vi "Inst_CNT90.vi"(8 "error in":errorcluster, 10 "All Message Queues in":T2, 11 "Prueba031 in":refnum<class "Prueba031.lvclass">) -> (0 "error out":errorcluster)   [LabVIEW 2019, in "Prueba031.lvclass"]
uses:
  Prueba031.lvclass
  QMH/Message Queue/All Message Queues.ctl
  QMH/Message Queue/Message Cluster.ctl
  Prueba031.lvclass/Prueba031.ctl
  <vilib>/Utility/error.llb/Error Cluster From Error Code.vi
  QMH/Message Queue/Enqueue Message (Single).vi
  <vilib>/ErrorRing/Error Ring.xnode
  QMH/Message Queue/Message Queue.lvlib
  Instrumento/CNT90/CNT90.lvclass
panel:
  out "elements":T1[](array[typedef])
  out "# elements in queue":i32
  out "K_iter":i32
  out "All States":string[](array[string])
  out "Actual State":string
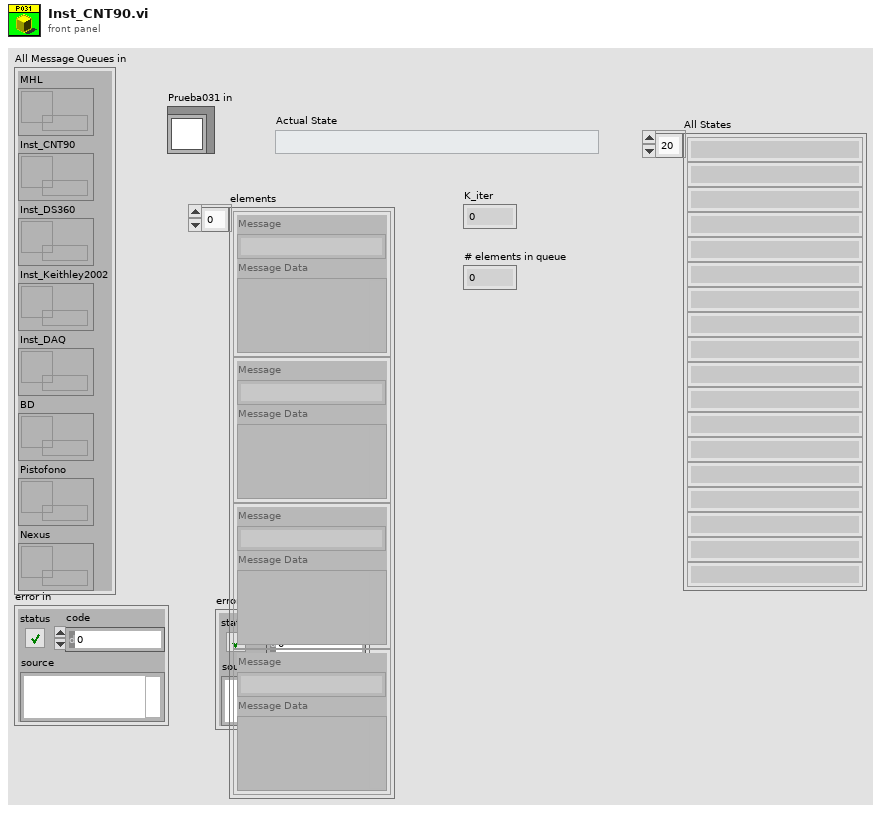
[diagram p1: front panel]
types:
  T1 = typedef "Message Queue.lvlib/Message Cluster.ctl" = cluster{"Message":string, "Message Data":variant}
  T2 = typedef "Message Queue.lvlib/All Message Queues.ctl" = cluster{"MHL":refnum<queue>, "Inst_CNT90":refnum<queue>, "Inst_DS360":refnum<queue>, "Inst_Keithley2002":refnum<queue>, "Inst_DAQ":refnum<queue>, "BD":refnum<queue>, "Pistofono":refnum<queue>, "Nexus":refnum<queue>}
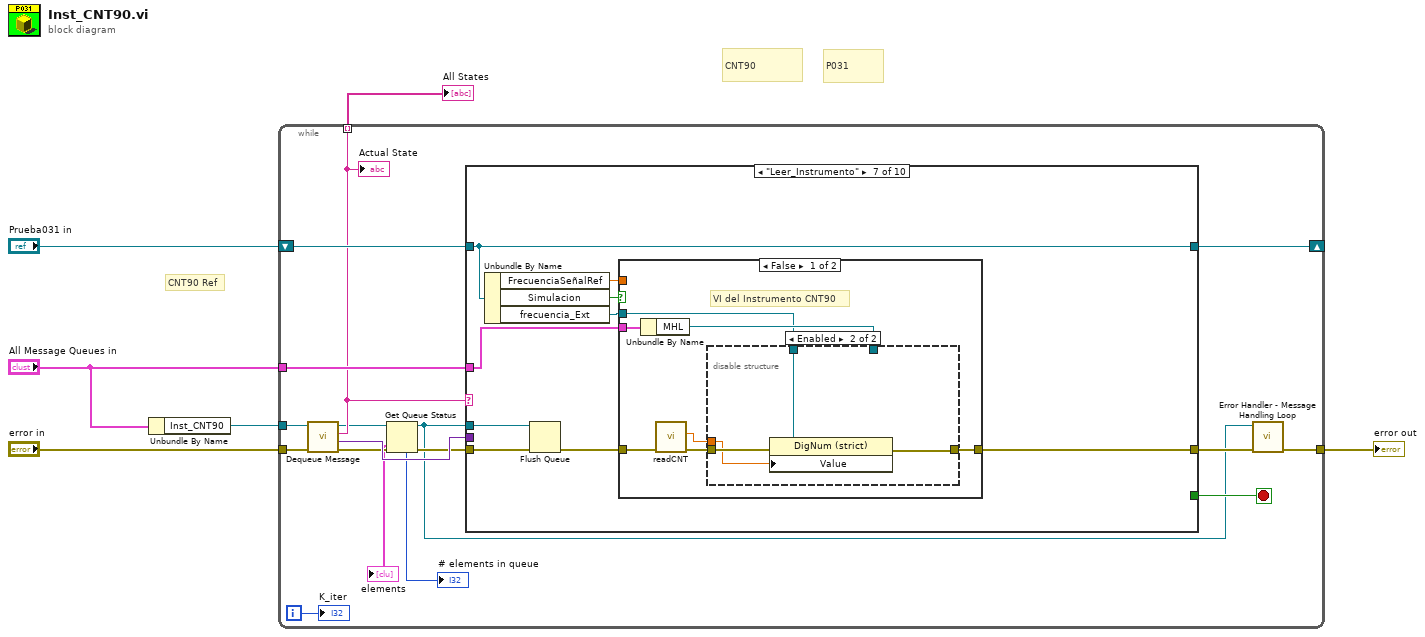
[diagram p0: block diagram]
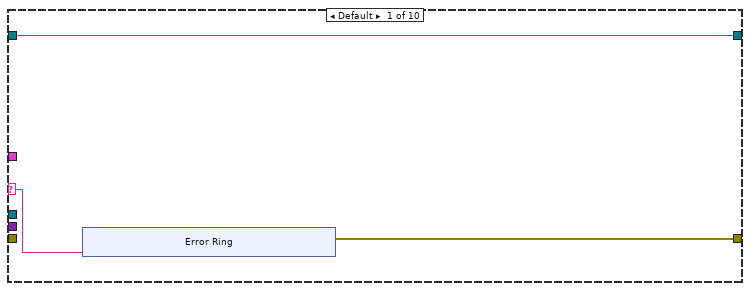
[diagram p2: hidden frame]
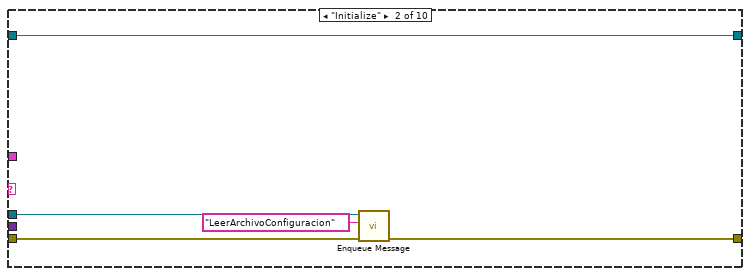
[diagram p3: hidden frame]
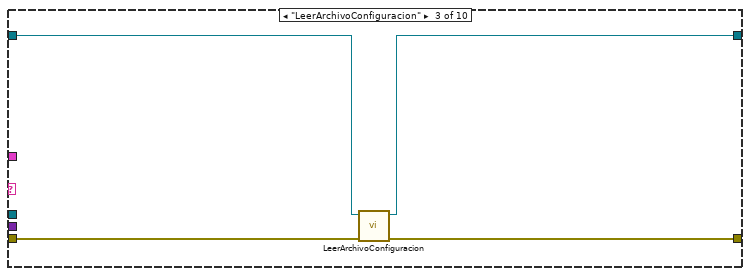
[diagram p4: hidden frame]
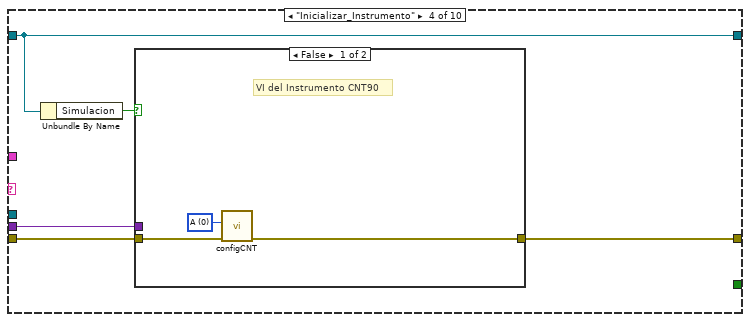
[diagram p5: hidden frame]
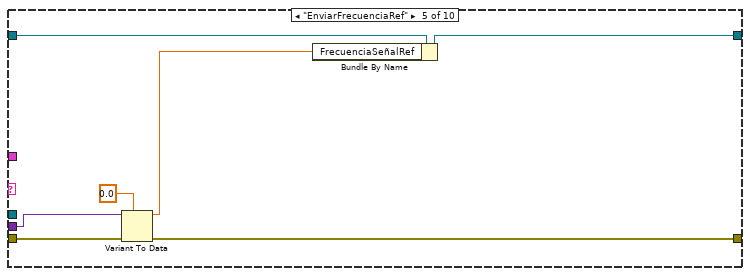
[diagram p7: hidden frame]
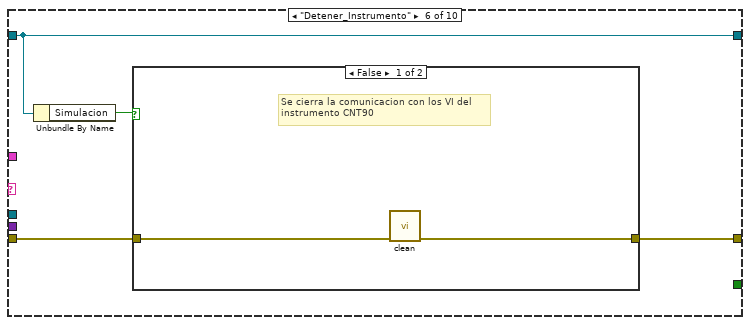
[diagram p8: hidden frame]
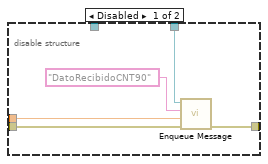
[diagram p10: hidden frame]
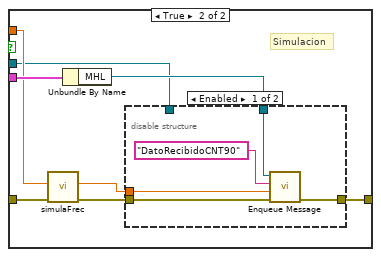
[diagram p11: hidden frame]
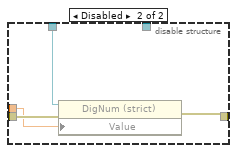
[diagram p12: hidden frame]
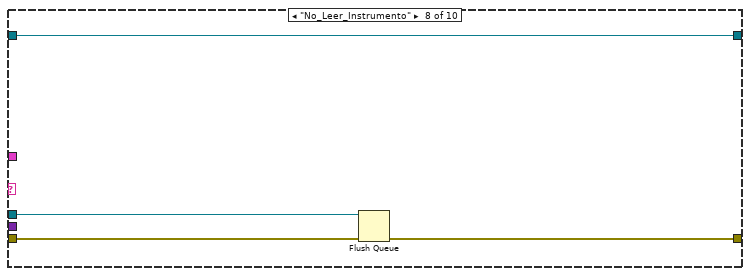
[diagram p13: hidden frame]
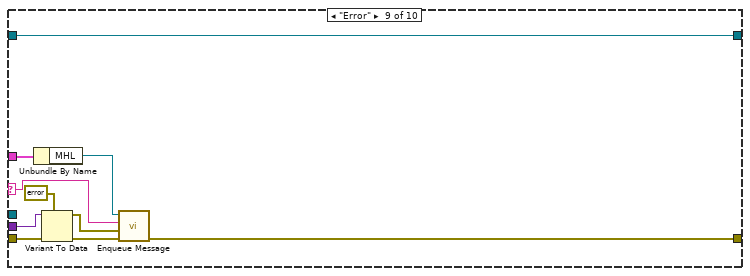
[diagram p14: hidden frame]
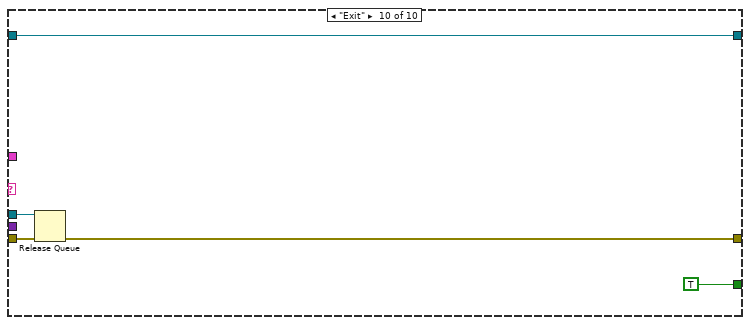
[diagram p15: hidden frame]
diagram:
  # "P031"
  # "CNT90"
  # "CNT90 Ref"
  n1 = Unbundle By Name("All Message Queues in") -> ("Inst_CNT90"=w5:refnum<queue>)
  n2 = while {
    tunnel: "error in" -> [w23]
    tunnel: w5 -> [w22]
    tunnel: "All Message Queues in" -> [w21]
    tunnel: [w14] -> w3
    shift-right: [w17] -> _
    shift-left: "Prueba031 in" -> [w20]
    tunnel: [w13] -> w2 mode=indexing
    i -> [w12]
    stop <- w16 stop-if-true
    n3 = call "Dequeue Message.vi"("error in (no error)"=w23, "Message Queue"=w22) -> ("error out"=w18:errorcluster, "Message Data"=w19:variant, "Message"=w13:string, "dup Message Queue"=w10:refnum<queue>)  [unwired: 6 in]
    "Actual State" <- w13
    n4 = Get Queue Status(queue=w10, error in (no error)=w18) -> (queue out=w9:refnum<queue>, error out=w11:errorcluster, # elements in queue=→"# elements in queue":i32, elements=→"elements":T1[])  [unwired: 1 in, 4 out]
    n5 = case shown="\"Leer_Instrumento\"" w13 {
      selector: w13 -> [w26 _ _ _ _ _ _ _ w116 _]
      tunnel: w21 -> [_ _ _ _ _ _ w70 _ w115 _]
      tunnel: w20 -> [w24 w38 w40 w47 w57 w61 w72 w110 w113 w123]
      tunnel: w9 -> [_ w35 _ _ _ _ w66 w108 _ w125]
      tunnel: w19 -> [_ _ _ w43 w54 _ _ _ w119 _]
      tunnel: w11 -> [_ w37 w42 w46 w58 w59 w74 w111 w120 w126]
      tunnel: [w25 w36 w41 w44 w55 w62 w73 w109 w112 w122] -> w15
      tunnel: [w24 w38 w39 w47 w56 w61 w72 w110 w113 w123] -> w17
      tunnel: [_ _ _ _ _ _ _ _ _ TRUE] -> w16
      frame Default {
        n6 = xnode "Error Ring"("parameter 0"=w26) -> ("error out"=w25:errorcluster)
      }
      frame "Initialize" {
        n7 = call-poly "Enqueue Message.vi"("error in (no error)"=w37, "Message"="LeerArchivoConfiguracion", "Message Queue"=w35) -> ("error out"=w36:errorcluster)  [unwired: 7 in, 1 out]
      }
      frame "LeerArchivoConfiguracion" {
        n8 = call "LeerArchivoConfiguracion.vi"("error in"=w42, "Prueba31 in"=w40) -> ("error out"=w41:errorcluster, "Prueba31 out"=w39:refnum<class "Prueba031.lvclass">)  [unwired: 8 in]
      }
      frame "Inicializar_Instrumento" {
        n9 = Unbundle By Name(w47) -> ("Simulacion"=w45:bool)
        n10 = case shown="False" w45 {
          tunnel: [w50 w51] -> w44
          tunnel: w46 -> [w49 w51]
          tunnel: w43 -> [_ _]
          frame False {
            w48 = 0 items=["A", "B"] ("Channel  1")
            # "VI del Instrumento CNT90"
            n11 = call "configCNT.vi"("error in (no error)"=w49, "Channel  1"=w48) -> ("error out"=w50:errorcluster)  [unwired: 8 in, 1 out]
          }
          frame True {
            # "Simulacion"
          }
        }
      }
      frame "EnviarFrecuenciaRef" {
        n12 = Variant To Data(error in=w58, type=0.0 ("FrecuenciaSeñalRef"), Variant=w54) -> (data=w52:dbl, error out=w55:errorcluster)
        n13 = Bundle By Name(cluster=w57, "FrecuenciaSeñalRef"=w52) -> (w56:refnum<class "Prueba031.lvclass">)
      }
      frame "Detener_Instrumento" {
        n14 = Unbundle By Name(w61) -> ("Simulacion"=w60:bool)
        n15 = case shown="False" w60 {
          tunnel: [w64 w65] -> w62
          tunnel: w59 -> [w63 w65]
          frame False {
            # "Se cierra la comunicacion con los VI del\ninstrumento CNT90"
            n16 = call "clean.vi"("error in (no error)"=w63) -> ("error out"=w64:errorcluster)  [unwired: 9 in, 1 out]
          }
          frame True {
            # "Simulacion"
          }
        }
      }
      frame "Leer_Instrumento" {
        n17 = Unbundle By Name(w72) -> ("FrecuenciaSeñalRef"=w69:dbl, "Simulacion"=w71:bool, "frecuencia_Ext"=w68:refnum<vi>)
        n18 = Flush Queue(queue=w66, error in (no error)=w74) -> (error out=w67:errorcluster)  [unwired: 2 out]
        n19 = case shown="False" w71 {
          tunnel: [w79 w98] -> w73
          tunnel: w67 -> [w81 w95]
          tunnel: w70 -> [w78 w97]
          tunnel: w69 -> [_ w92]
          tunnel: w68 -> [w75 w91]
          frame False {
            # "VI del Instrumento CNT90"
            n20 = Unbundle By Name(w78) -> ("MHL"=w77:refnum<queue>)
            n21 = call "readCNT.vi"("error in (no error)"=w81) -> ("error out"=w80:errorcluster, "medicion"=w76:dbl)  [unwired: 8 in, 1 out]
            n22 = disable-structure shown="Enabled" {
              disable-tunnel: w80 -> [w85 w90]
              disable-tunnel: [w84 w89] -> w79
              disable-tunnel: w77 -> [w83 _]
              disable-tunnel: w76 -> [w82 w87]
              disable-tunnel: w75 -> [_ w88]
              frame Disabled {
                n23 = call-poly "Enqueue Message.vi"("error in (no error)"=w85, "Message Data"=w82, "Message"="DatoRecibidoCNT90", "Message Queue"=w83) -> ("error out"=w84:errorcluster)  [unwired: 6 in, 1 out]
              }
              frame Enabled {
                n24 = property class="DigNum (strict)"(reference=w88, error in=w90, "Value"=w87) -> (error out=w89:errorcluster)  [unwired: 1 out]
              }
            }
          }
          frame True {
            # "Simulacion"
            n25 = call "simulaFrec.vi"("error in (no error)"=w95, "frec in"=w92) -> ("error out"=w94:errorcluster, "frec out"=w93:dbl)  [unwired: 7 in, 1 out]
            n26 = Unbundle By Name(w97) -> ("MHL"=w96:refnum<queue>)
            n27 = disable-structure shown="Enabled" {
              disable-tunnel: [w102 w106] -> w98
              disable-tunnel: w96 -> [w101 _]
              disable-tunnel: w94 -> [w100 w107]
              disable-tunnel: w93 -> [w99 w104]
              disable-tunnel: w91 -> [_ w105]
              frame Enabled {
                n28 = call-poly "Enqueue Message.vi"("error in (no error)"=w100, "Message Data"=w99, "Message"="DatoRecibidoCNT90", "Message Queue"=w101) -> ("error out"=w102:errorcluster)  [unwired: 6 in, 1 out]
              }
              frame Disabled {
                n29 = property class="DigNum (strict)"(reference=w105, error in=w107, "Value"=w104) -> (error out=w106:errorcluster)  [unwired: 1 out]
              }
            }
          }
        }
      }
      frame "No_Leer_Instrumento" {
        n30 = Flush Queue(queue=w108, error in (no error)=w111) -> (error out=w109:errorcluster)  [unwired: 2 out]
      }
      frame "Error" {
        n31 = Unbundle By Name(w115) -> ("MHL"=w114:refnum<queue>)
        n32 = Variant To Data(error in=w120, type=errorcluster {"status"=FALSE, "code"=0, "source"=""} ("error constant"), Variant=w119) -> (data=w117:errorcluster, error out=w118:errorcluster)
        n33 = call-poly "Enqueue Message.vi"("error in (no error)"=w118, "Message Data"=w117, "Message"=w116, "Message Queue"=w114) -> ("error out"=w112:errorcluster)  [unwired: 6 in, 1 out]
      }
      frame "Exit" {
        n34 = Release Queue(queue=w125, error in (no error)=w126) -> (error out=w122:errorcluster)  [unwired: 1 in, 2 out]
      }
    }
    n35 = call "Error Handler - Message Handling Loop.vi"("error in (no error)"=w15, "Message Queue"=w9) -> ("dup error in"=w14:errorcluster)  [unwired: 8 in, 1 out]
    "K_iter" <- w12
  }
  "error out" <- w3
  "All States" <- w2
